vi "enqueue_states.vi"(6 "task":T1=[enum."(qsm) initialize"], 7 "error in":errorcluster, 10 "queue in":refnum<queue>) -> (0 "error out":errorcluster, 3 "queue out":refnum<queue>)   [LabVIEW 2017]
uses:
  type defs/states.ctl
  type defs/task.ctl
panel:
  # "enqueue_states"
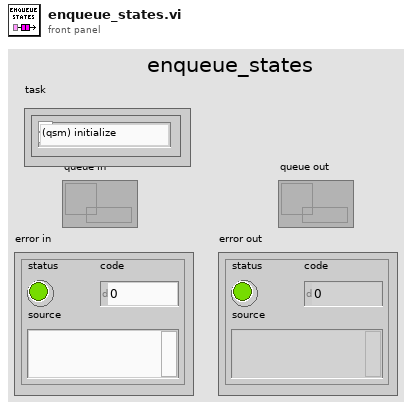
[diagram p1: front panel]
types:
  T1 = typedef "task.ctl" = T2[]
  T2 = typedef "states.ctl" = enum16{"(qsm) schedule", "(qsm) initialize", "(qsm) release", "(qsm) clean up", "(qsm) shutdown", "(myRIO) initialize", "(myRIO) clean up", "(myRIO) update ports", "Setup get", "(image) get", "(image) show", "(ball) Shape detection", "(ball) Calc ball indx", "(ball) Calculate ROI", "(ball) Analyze color", "(ball) Align", "(ball) Wait", "(ball) Grab", "(pattern) Find Square", "(pattern) Calculate ROI", "(pattern) Calc pattern indx", "Compare", "(pattern) Analyze pattern", "(pattern) Align", "(pattern) Wait", "(pattern) states control", "navx", "stop motors", "(joystick) Joystick control", "_Timer", "Setup manipulator", "(auto) Count balls", "(auto) Analyze balls", "(auto) Dot Controller", "(auto) Fwd (cm)", "(auto) Turn (angle)", "(auto) Tnl (M2-M2.5)", "(auto) Recover Def Pos", "(auto) Go Back Controller", "Wait for button"}
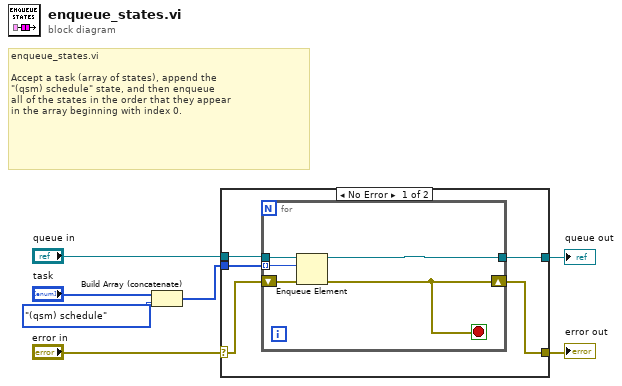
[diagram p0: block diagram]
diagram:
  # "enqueue_states.vi\n\nAccept a task (array of states), append the\n\"(qsm) schedule\" state, and then enqueue\nall of the states in the order that they appear\nin the array beginning with index 0."
  n1 = Build Array (concatenate) "Build Array"("task", states."(qsm) schedule" ("element")) -> (w2:T1)
  n2 = case shown="No Error" "error in" {
    selector: "error in" -> [w10 w19]
    tunnel: [w9 w19] -> w6
    tunnel: "queue in" -> [w12 w18]
    tunnel: [w11 w18] -> w4
    tunnel: w2 -> [w8 _]
    frame No Error {
      n3 = for {
        shift-right: [w14] -> w9
        shift-left: w10 -> [w17]
        tunnel: w12 -> [w16]
        tunnel: w8 -> [w15] mode=indexing
        tunnel: [w13] -> w11
        stop <- w14 stop-if-true
        n4 = Enqueue Element(queue=w16, element=w15, error in (no error)=w17) -> (queue out=w13:refnum<queue>, error out=w14:errorcluster)  [unwired: 1 in, 1 out]
      }
    }
    frame Error {
    }
  }
  "queue out" <- w4
  "error out" <- w6
